vi "1.5.vi"() -> ()   [LabVIEW 2013]
panel:
  in  "Boolean":bool
  out "Temperatura Convertida":dbl caption="[c]"
  in  "Temperatura a Convertir":dbl caption="F"
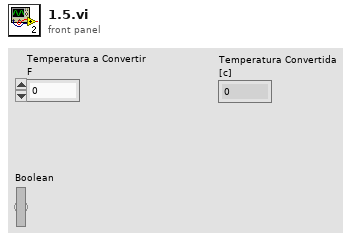
[diagram p1: front panel]
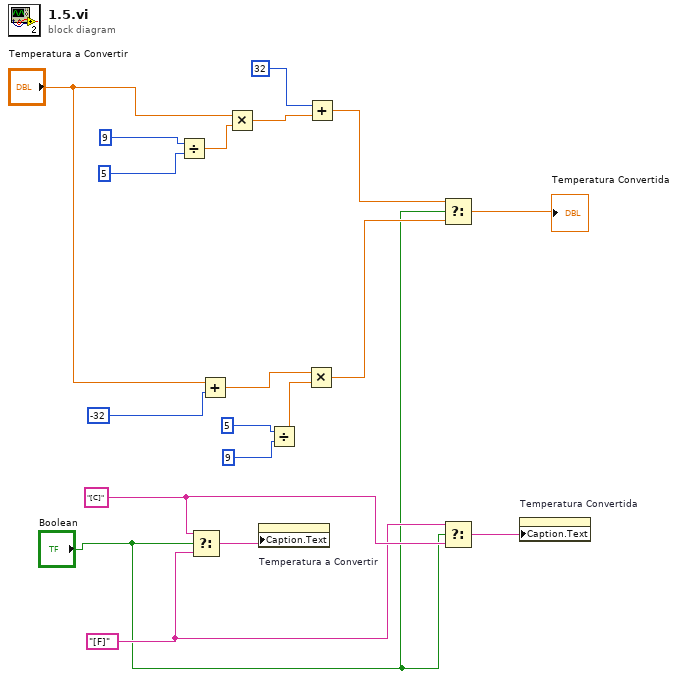
[diagram p0: block diagram]
diagram:
  w3 = "[F]"
  w4 = "[C]"
  n1 = Divide(x=9, y=5) -> (x/y=w9:dbl)
  n2 = Select(t=w4, s="Boolean", f=w3) -> (s? t:f=w5:string)
  n3 = Add(x="Temperatura a Convertir", y=-32) -> (x+y=w18:dbl)
  n4 = Multiply(x="Temperatura a Convertir", y=w9) -> (x*y=w11:dbl)
  n5 = property on="Temperatura a Convertir" class="DigNum (strict)"("Caption.Text"=w5) -> ()  [unwired: 2 in, 2 out]
  n6 = Divide(x=5, y=9) -> (x/y=w15:dbl)
  n7 = Multiply(x=w18, y=w15) -> (x*y=w7:dbl)
  n8 = Add(x=32, y=w11) -> (x+y=w8:dbl)
  n9 = Select(t=w8, s="Boolean", f=w7) -> (s? t:f=→"Temperatura Convertida":dbl)
  n10 = Select(t=w3, s="Boolean", f=w4) -> (s? t:f=w2:string)
  n11 = property on="Temperatura Convertida" class="DigNum (strict)"("Caption.Text"=w2) -> ()  [unwired: 2 in, 2 out]
